vi "BottomStacking.vi"(7 "Cancel Button":bool, 10 "Activating Button":bool) -> ()   [LabVIEW 2014]
uses:
  2015 Main Project/BottomStacking.ctl
  2015 Main Project/Robot Global Data.vi
  <vilib>/Rock Robotics/WPI/RobotDrive/WPI_RobotDriveGetSetRefNum.vi
  <vilib>/Rock Robotics/WPI/RobotDrive/WPI_RobotDriveArcadeDrive_Standard(NoSaturation).vi
panel:
  in  "Tote Num Get":dbl
  out "Drive Motors Set":dbl
  out "End Effector Set":dbl
  out "Tote Number":dbl
  out "Ejector Motor Set":dbl
  in  "Winch Sensor Position":dbl
  out "Winch Cims Setpoint":dbl
  in  "Ejector Encoder Rate":dbl
  out "State Machine":T1
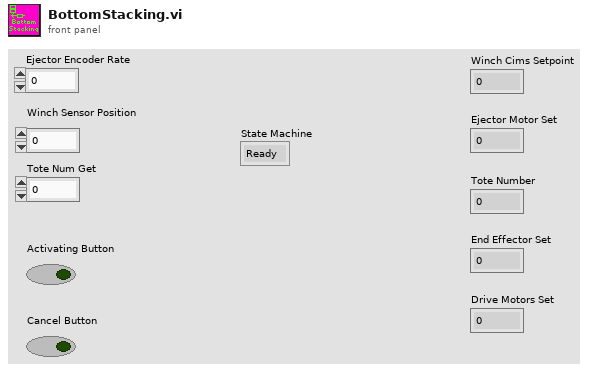
[diagram p1: front panel]
types:
  T1 = typedef "BottomStacking.ctl" = enum16{"Ready", "Raise To Stack Height", "Eject Internal Stack", "Set Down On Stack", "Release Tote", "Back Away", "Reset", "Emergency Stop"}
  T2 = typedef "WPI_EncoderDevRef.ctl" = cluster{"DevStatus":errorcluster, "EncoderIndex":T3, "CounterIndex":T4, "DistancePerCount":dbl, "Decoding Type":T5}
  T3 = typedef "FPGA_EncoderIdx.ctl" = enum8{"Enc 0", "Enc 1", "Enc 2", "Enc 3", "Enc 4", "Enc 5", "Enc 6", "Enc 7", "Invalid"}
  T4 = typedef "FPGA_CounterCtrSystemIndex.ctl" = enum8{"Ctr 0", "Ctr 1", "Ctr 2", "Ctr 3", "Ctr 4", "Ctr 5", "Ctr 6", "Ctr 7", "Invalid"}
  T5 = typedef "WPI_EncoderType.ctl" = enum16{"1x", "2x", "4x"}
  T6 = typedef "WPI_MotorControlDeviceRef.ctl" = cluster{"DeviceStatus":errorcluster, "Type":T7, "PWM":cluster{"Controller":T8, "PWM Channel":T9, "DeadBand":T10}, "CAN":cluster{"Device Number":u8, "Control Mode":T11, "Semaphore":T12, "Max Vout":dbl, "TalonSRX Control Mode":T13}, "Invert":bool, "TransformRef":T14, "InvTransformRef":T14}
  T7 = typedef "WPI_MotorControlType.ctl" = enum16{"PWM", "CAN", "CANTalonSRX"}
  T8 = typedef "FPGA_TypedefDigitalModule.ctl" = enum16{"Controller 1"}
  T9 = typedef "FPGA_DIOPWMChannel.ctl" = enum8{"PWM 0", "PWM 1", "PWM 2", "PWM 3", "PWM 4", "PWM 5", "PWM 6", "PWM 7", "PWM 8", "PWM 9", "PWM MXP 0", "PWM MXP 1", "PWM MXP 2", "PWM MXP 3", "PWM MXP 4", "PWM MXP 5", "PWM MXP 6", "PWM MXP 7", "PWM MXP 8", "PWM MXP 9", "Invalid"}
  T10 = typedef "WPI_PWMDeadband.ctl" = cluster{"Name":string, "maxPositivePwm":i32, "minPositivePwm":i32, "centerPwm":i32, "maxNegativePwm":i32, "minNegativePwm":i32, "angularRange":u16}
  T11 = typedef "WPI_CANJaguar_ControlMode.ctl" = enum8{"Percent VBus", "Current", "Speed", "Position", "Voltage"}
  T12 = typedef "Semaphore RefNum" = refnum<k1>
  T13 = typedef "WPI_CANTalonSRX_APIControlMode.ctl" = enum8{"Percent VBus", "Speed", "Position", "Slave", "Unchanged / Invalid"}
  T14 = typedef "WPI_PWMTransform_ConPane.ctl" = refnum<vi>
  T15 = typedef "WPI_CANTalonSRX_GlobalStatus.ctl" = cluster{"Applied Throttle":dbl, "Module Enabled":bool, "CAN Error":errorcluster, "Closed Loop Error":dbl, "Forward Limit Switch Closed":bool, "Reverse Limit Switch Closed":bool, "Sensor Position":dbl, "Sensor Velocity":dbl, "Current":dbl, "Sticky Fault - Over Temp":bool, "Sticky Fault - Under Voltage":bool, "Sticky Fault - Forward Limit":bool, "Sticky Fault - Reverse Limit":bool, "Sticky Fault - Forward Soft Limit":bool, "Sticky Fault - Reverse Soft Limit":bool, "Brake is Enabled":bool, "Encoder Position":dbl, "Encoder Velocity":dbl, "Encoder Index Count":dbl, "Encoder A Pin State":bool, "Encoder B Pin State":bool, "Encoder Index Pin State":bool, "Analog In":dbl, "Analog In Velocity":dbl, "Temperature (C)":dbl, "Battery Voltage":dbl}
  T16 = typedef "WPI_RobotDriveDevRef.ctl" = cluster{"DevStatus":errorcluster, "Motors[]":T6[], "Square Inputs":bool, "Max Output":dbl}
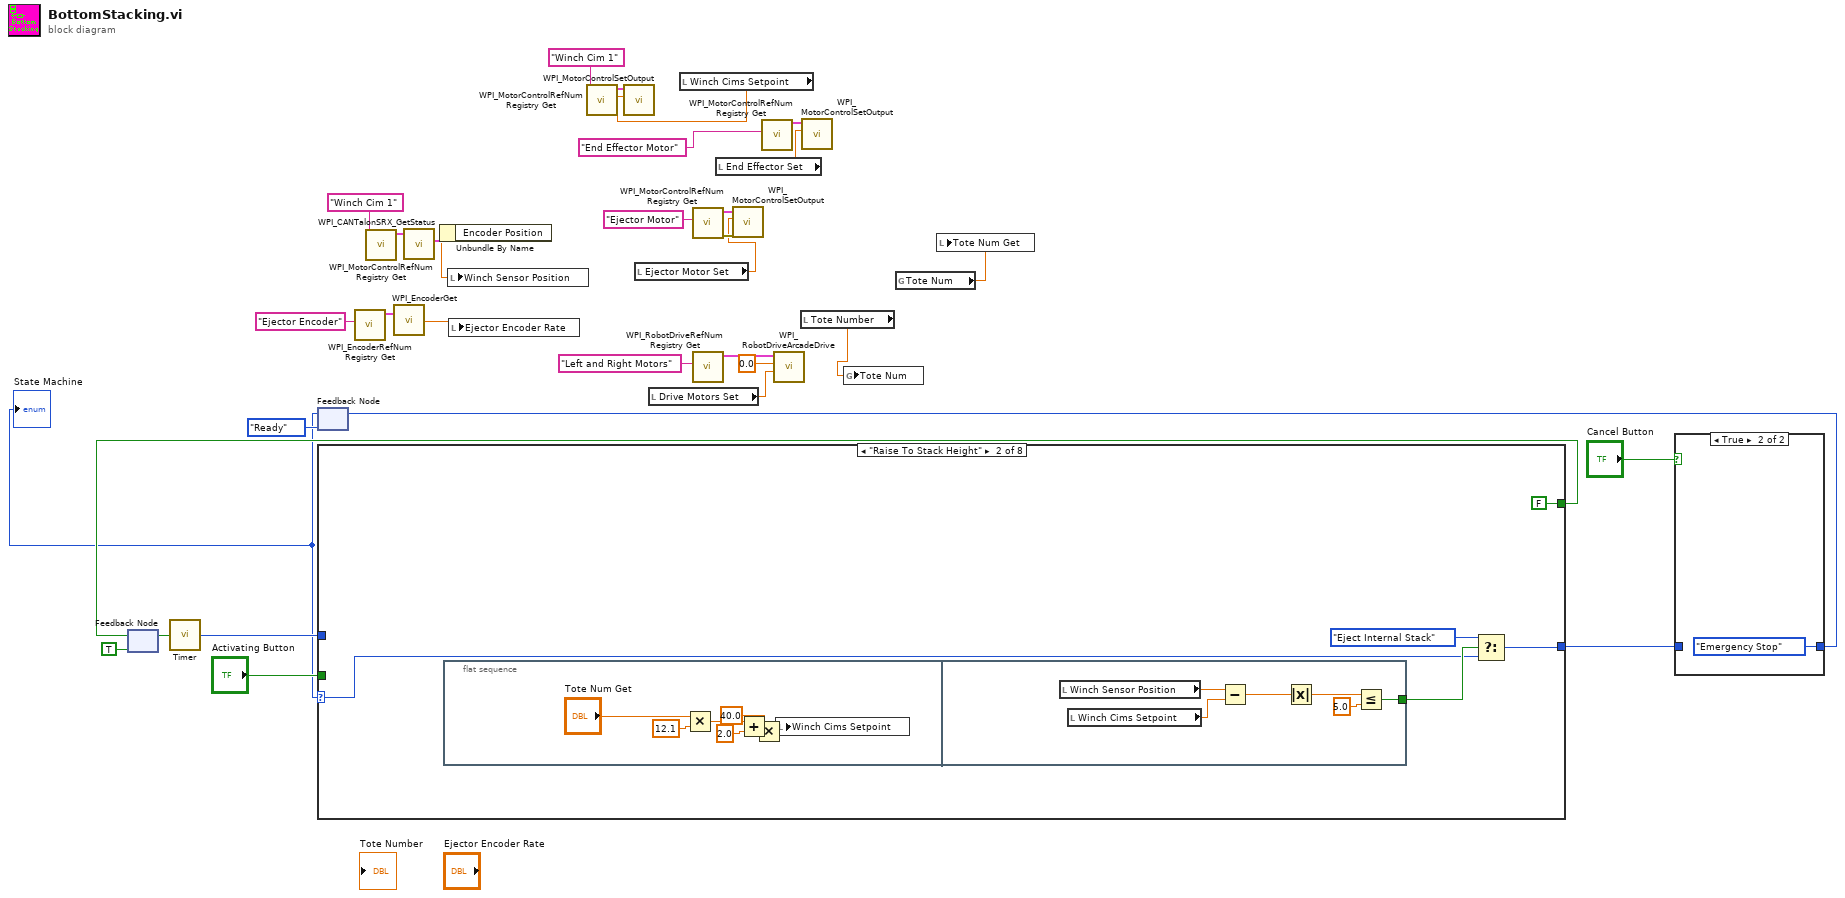
[diagram p0: block diagram]
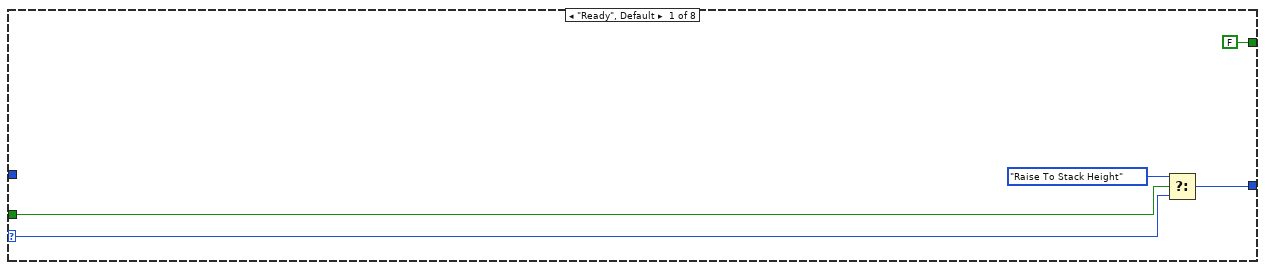
[diagram p3: hidden frame]
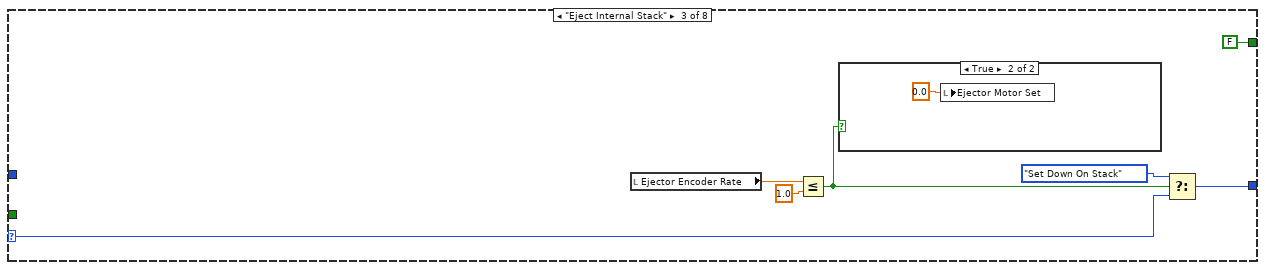
[diagram p4: hidden frame]
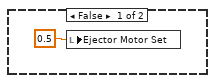
[diagram p5: hidden frame]
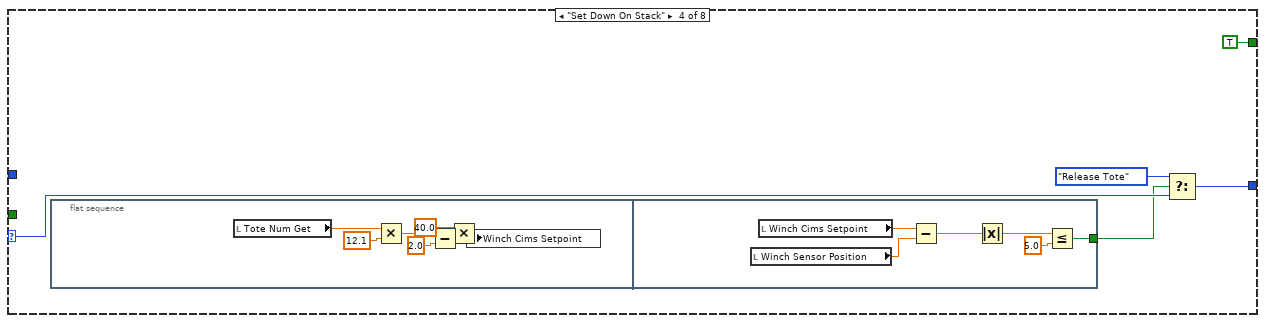
[diagram p6: hidden frame]
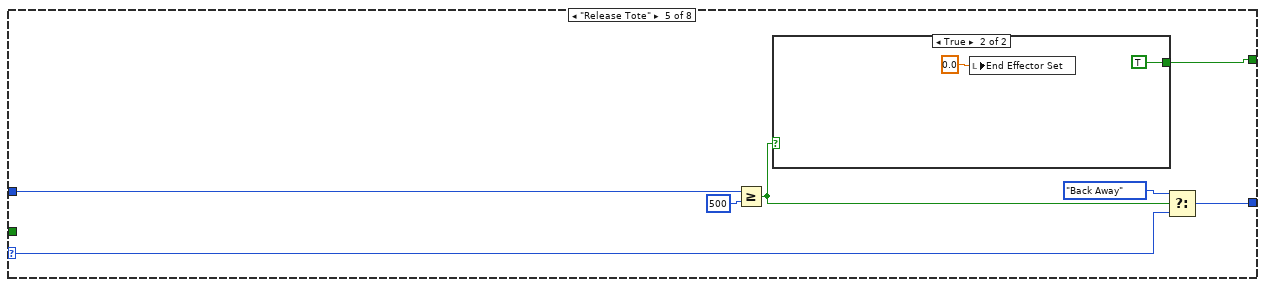
[diagram p7: hidden frame]
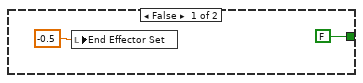
[diagram p8: hidden frame]
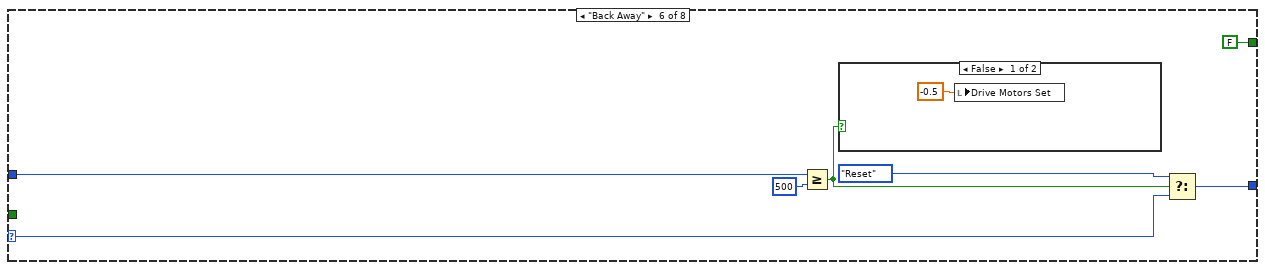
[diagram p9: hidden frame]
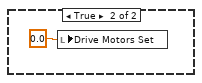
[diagram p10: hidden frame]
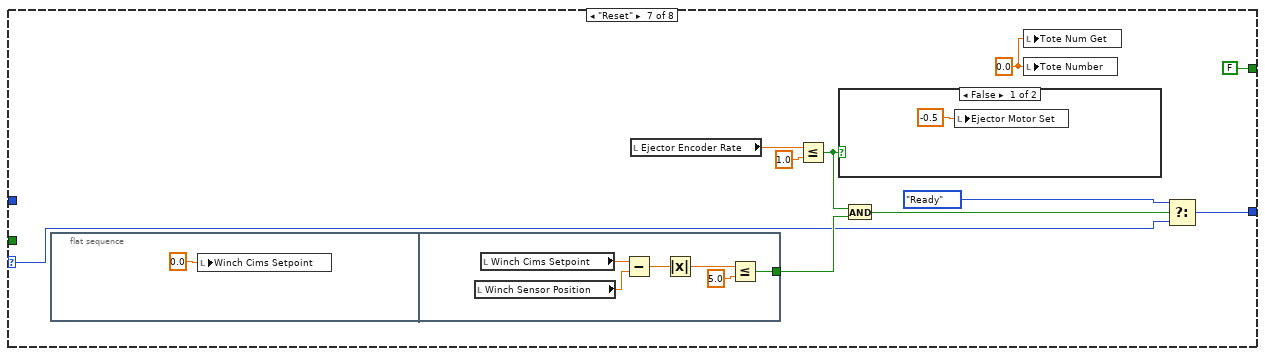
[diagram p11: hidden frame]
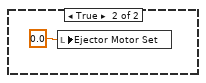
[diagram p12: hidden frame]
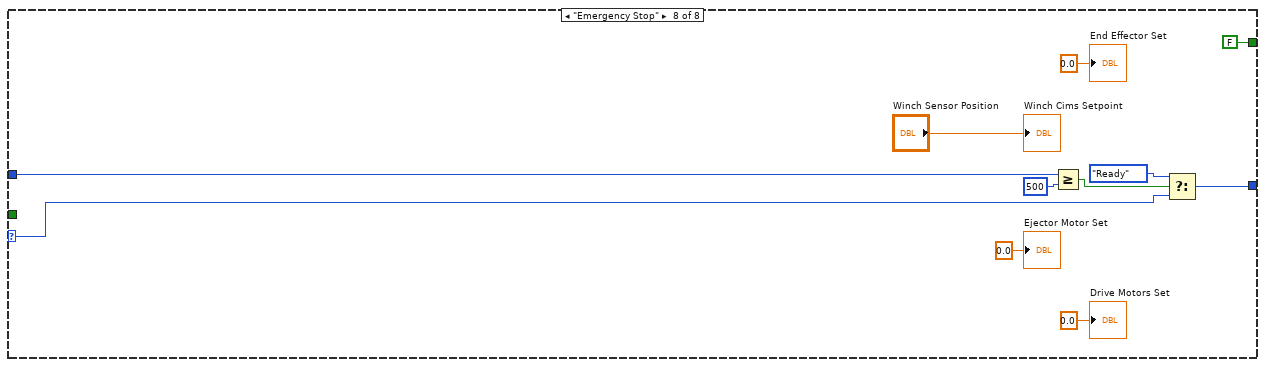
[diagram p13: hidden frame]
diagram:
  n1 = feedback #1(TRUE) -> (w31:bool)
  n2 = call "Timer.vi"("Set Timer"=w31) -> ("Time elapsed"=w29:u64)
  n3 = feedback #2(BottomStacking."Ready" ("State Machine")) -> (w24:T1)
  "State Machine" <- w24
  n4 = case shown="\"Raise To Stack Height\"" w24 {
    selector: w24 -> [w34 w39 w62 w69 w90 w97 w107 w129]
    tunnel: "Activating Button" -> [w38 _ _ _ _ _ _ _]
    tunnel: [w36 w43 w63 w70 w89 w95 w113 w127] -> w26
    tunnel: [FALSE FALSE FALSE TRUE w84 FALSE FALSE FALSE] -> w30
    tunnel: w29 -> [_ _ _ _ w87 w100 _ w131]
    frame "Ready", Default {
      n5 = Select(t=BottomStacking."Raise To Stack Height" ("State Machine"), s=w38, f=w34) -> (s? t:f=w36:T1)
    }
    frame "Raise To Stack Height" {
      n6 = flat-sequence {
        tunnel: [w51] -> w40
        frame #0 {
          n7 = Multiply(x="Tote Num Get", y=12.1) -> (x*y=w48:dbl)
          n8 = Add(x=w48, y=2.0) -> (x+y=w50:dbl)
          n9 = Multiply(x=w50, y=40.0) -> (x*y=w45:dbl)
          n10 = local write "Winch Cims Setpoint"(w45) -> ()
        }
        frame #1 {
          n11 = local read "Winch Sensor Position"() -> (w55:dbl)
          n12 = local read "Winch Cims Setpoint"() -> (w56:dbl)
          n13 = Subtract(x=w55, y=w56) -> (x-y=w52:dbl)
          n14 = Absolute Value(x=w52) -> (abs(x)=w53:dbl)
          n15 = Less Or Equal?(x=w53, y=5.0) -> (x <= y?=w51:bool)
        }
      }
      n16 = Select(t=BottomStacking."Eject Internal Stack" ("State Machine"), s=w40, f=w39) -> (s? t:f=w43:T1)
    }
    frame "Eject Internal Stack" {
      n17 = local read "Ejector Encoder Rate"() -> (w59:dbl)
      n18 = Less Or Equal?(x=w59, y=1.0) -> (x <= y?=w57:bool)
      n19 = case shown="True" w57 {
        frame False {
          n20 = local write "Ejector Motor Set"(0.5 ("Ejector Motor Set")) -> ()
        }
        frame True {
          n21 = local write "Ejector Motor Set"(0.0 ("Ejector Motor Set")) -> ()
        }
      }
      n22 = Select(t=BottomStacking."Set Down On Stack" ("State Machine"), s=w57, f=w62) -> (s? t:f=w63:T1)
    }
    frame "Set Down On Stack" {
      n23 = flat-sequence {
        tunnel: [w78] -> w66
        frame #0 {
          n24 = local read "Tote Num Get"() -> (w76:dbl)
          n25 = Multiply(x=w76, y=12.1 ("Elevator Setpoint")) -> (x*y=w74:dbl)
          n26 = Subtract(x=w74, y=2.0) -> (x-y=w77:dbl)
          n27 = Multiply(x=40.0, y=w77) -> (x*y=w72:dbl)
          n28 = local write "Winch Cims Setpoint"(w72) -> ()
        }
        frame #1 {
          n29 = local read "Winch Sensor Position"() -> (w79:dbl)
          n30 = local read "Winch Cims Setpoint"() -> (w80:dbl)
          n31 = Subtract(x=w80, y=w79) -> (x-y=w81:dbl)
          n32 = Absolute Value(x=w81) -> (abs(x)=w82:dbl)
          n33 = Less Or Equal?(x=w82, y=5.0) -> (x <= y?=w78:bool)
        }
      }
      n34 = Select(t=BottomStacking."Release Tote" ("State Machine"), s=w66, f=w69) -> (s? t:f=w70:T1)
    }
    frame "Release Tote" {
      n35 = Greater Or Equal?(x=w87, y=u64 500) -> (x >= y?=w85:bool)
      n36 = case shown="True" w85 {
        tunnel: [FALSE TRUE] -> w84
        frame False {
          n37 = local write "End Effector Set"(-0.5 ("Output")) -> ()
        }
        frame True {
          n38 = local write "End Effector Set"(0.0 ("Output")) -> ()
        }
      }
      n39 = Select(t=BottomStacking."Back Away" ("State Machine"), s=w85, f=w90) -> (s? t:f=w89:T1)
    }
    frame "Back Away" {
      n40 = Greater Or Equal?(x=w100, y=u64 500) -> (x >= y?=w98:bool)
      n41 = case shown="False" w98 {
        frame False {
          n42 = local write "Drive Motors Set"(-0.5 ("Y axis value")) -> ()
        }
        frame True {
          n43 = local write "Drive Motors Set"(0.0) -> ()
        }
      }
      n44 = Select(t=BottomStacking."Reset" ("State Machine"), s=w98, f=w97) -> (s? t:f=w95:T1)
    }
    frame "Reset" {
      w105 = 0.0 ("Tote Num")
      n45 = flat-sequence {
        tunnel: [w115] -> w108
        frame #0 {
          n46 = local write "Winch Cims Setpoint"(0.0 ("Ejector Motor Set")) -> ()
        }
        frame #1 {
          n47 = local read "Winch Sensor Position"() -> (w120:dbl)
          n48 = local read "Winch Cims Setpoint"() -> (w119:dbl)
          n49 = Subtract(x=w119, y=w120) -> (x-y=w118:dbl)
          n50 = Absolute Value(x=w118) -> (abs(x)=w117:dbl)
          n51 = Less Or Equal?(x=w117, y=5.0) -> (x <= y?=w115:bool)
        }
      }
      n52 = local read "Ejector Encoder Rate"() -> (w109:dbl)
      n53 = Less Or Equal?(x=w109, y=1.0) -> (x <= y?=w106:bool)
      n54 = case shown="False" w106 {
        frame False {
          n55 = local write "Ejector Motor Set"(-0.5 ("Ejector Motor Set")) -> ()
        }
        frame True {
          n56 = local write "Ejector Motor Set"(0.0 ("Ejector Motor Set")) -> ()
        }
      }
      n57 = And(x=w106, y=w108) -> (x .and. y?=w111:bool)
      n58 = local write "Tote Num Get"(w105) -> ()
      n59 = local write "Tote Number"(w105) -> ()
      n60 = Select(t=BottomStacking."Ready" ("State Machine"), s=w111, f=w107) -> (s? t:f=w113:T1)
    }
    frame "Emergency Stop" {
      n61 = Greater Or Equal?(x=w131, y=u64 500) -> (x >= y?=w130:bool)
      n62 = Select(t=BottomStacking."Ready" ("State Machine"), s=w130, f=w129) -> (s? t:f=w127:T1)
      "Ejector Motor Set" <- 0.0 ("Ejector Motor Set")
      "Winch Cims Setpoint" <- "Winch Sensor Position"
      "End Effector Set" <- 0.0 ("End Effector Set")
      "Drive Motors Set" <- 0.0 ("Drive Motors Set")
    }
  }
  n63 = feedback-in #1(w30) -> ()
  n64 = call <vilib>:"WPI_EncoderRefNum Registry Get.vi"("refnum name"="Ejector Encoder") -> ("EncoderDevRef"=w13:T2)  [unwired: 9 in, 1 out]
  n65 = call <vilib>:"WPI_MotorControlRefNum Registry Get.vi"("refnum name"="Winch Cim 1") -> ("MotorControlDevRef"=w23:T6)  [unwired: 9 in, 1 out]
  n66 = call <vilib>:"WPI_EncoderGet.vi"("EncoderDevRef"=w13) -> ("Rate"=w12:dbl)  [unwired: 5 in, 5 out]
  n67 = call <vilib>:"WPI_CANTalonSRX_GetStatus.vi"("CAN Talon SRX Ref"=w23) -> ("Talon SRX Status"=w21:T15)  [unwired: 8 in, 2 out]
  n68 = Unbundle By Name(w21) -> ("Encoder Position"=w20:dbl)
  n69 = local write "Winch Sensor Position"(w20) -> ()
  n70 = local write "Ejector Encoder Rate"(w12) -> ()
  n71 = call <vilib>:"WPI_MotorControlRefNum Registry Get.vi"("refnum name"="Winch Cim 1") -> ("MotorControlDevRef"=w16:T6)  [unwired: 9 in, 1 out]
  n72 = local read "Ejector Motor Set"() -> (w5:dbl)
  n73 = local read "Drive Motors Set"() -> (w2:dbl)
  n74 = local read "Winch Cims Setpoint"() -> (w15:dbl)
  n75 = call <vilib>:"WPI_MotorControlSetOutput.vi"("Output"=w15, "MotorControlDevRef"=w16) -> ()  [unwired: 7 in, 3 out]
  n76 = call <vilib>:"WPI_MotorControlRefNum Registry Get.vi"("refnum name"="Ejector Motor") -> ("error out"=w6:errorcluster, "MotorControlDevRef"=w7:T6)  [unwired: 9 in]
  n77 = call <vilib>:"WPI_RobotDriveRefNum Registry Get.vi"("refnum name"="Left and Right Motors") -> ("RobotDriveDevRef"=w4:T16)  [unwired: 9 in, 1 out]
  n78 = local read "End Effector Set"() -> (w18:dbl)
  n79 = call <vilib>:"WPI_MotorControlSetOutput.vi"("error in (no error)"=w6, "Output"=w5, "MotorControlDevRef"=w7) -> ()  [unwired: 6 in, 3 out]
  n80 = call <vilib>:"WPI_MotorControlRefNum Registry Get.vi"("refnum name"="End Effector Motor") -> ("MotorControlDevRef"=w19:T6)  [unwired: 9 in, 1 out]
  n81 = call-poly <vilib>:"WPI_RobotDriveArcadeDrive.vi"("Y axis value"=w2, "X axis value"=0.0, "RobotDriveDevRef"=w4) -> ()  [unwired: 6 in, 3 out]
  n82 = local read "Tote Number"() -> (w11:dbl)
  n83 = call <vilib>:"WPI_MotorControlSetOutput.vi"("Output"=w18, "MotorControlDevRef"=w19) -> ()  [unwired: 7 in, 3 out]
  n84 = global write "Robot Global Data.vi" "Tote Num"(w11) -> ()
  n85 = global read "Robot Global Data.vi" "Tote Num"() -> (w10:dbl)
  n86 = local write "Tote Num Get"(w10) -> ()
  n87 = case shown="True" "Cancel Button" {
    tunnel: [w134 BottomStacking."Emergency Stop" ("State Machine")] -> w27
    tunnel: w26 -> [w134 _]
    frame False {
    }
    frame True {
    }
  }
  n88 = feedback-in #2(w27) -> ()
